vi "Test_Project Parser.vi"() -> ()   [LabVIEW 2019]
uses:
  Build/Project.Dependencies Finder.lvlibp/Dependency Source_VIPM/Dependency Source_VIPM.lvclass
  C:/Current projects/LV32.2019..ProjectDependenciesFinder/Build/Project.Dependencies Finder.lvlibp/Dependency Source/Dependency Source.lvclass
  Build/Project.Dependencies Finder.lvlibp/Dependency Source_NIPM/Dependency Source_NIPM.lvclass
  Build/Project.Dependencies Finder.lvlibp/Dependency Source_GPM/Dependency Source_GPM.lvclass
  Build/Project.Dependencies Finder.lvlibp/Dependency Source_Custom/Dependency Source_Custom.lvclass
  Build/Project.Dependencies Finder.lvlibp/Ctl/Ctl_Internal Target Element.ctl
  Build/Project.Dependencies Finder.lvlibp
  Build/Project.Dependencies Finder.lvlibp/Ctl/Ctl_External Target Element.ctl
  GPM/gpm_packages/@cs/actor-framework-messages/Source/MessageCycle/Message Cycle Notifications.ctl
  GPM/gpm_packages/@cs/actor-framework-messages/Source/MessageCycle/MessageCycle.lvclass
panel:
  in  "Load Stored Targets?(T)":bool=TRUE
  out "Unhandled Targets":string[](array[string])
  out "External Dependencies":string[](array[string])
  out "Internal Dependencies":string[](array[string])
  out "Error Out":errorcluster
  in  "Project Path in":path=path "C:/Current projects/LV32.2019..ProjectDependenciesFinder/_Test/Test.lvproj"
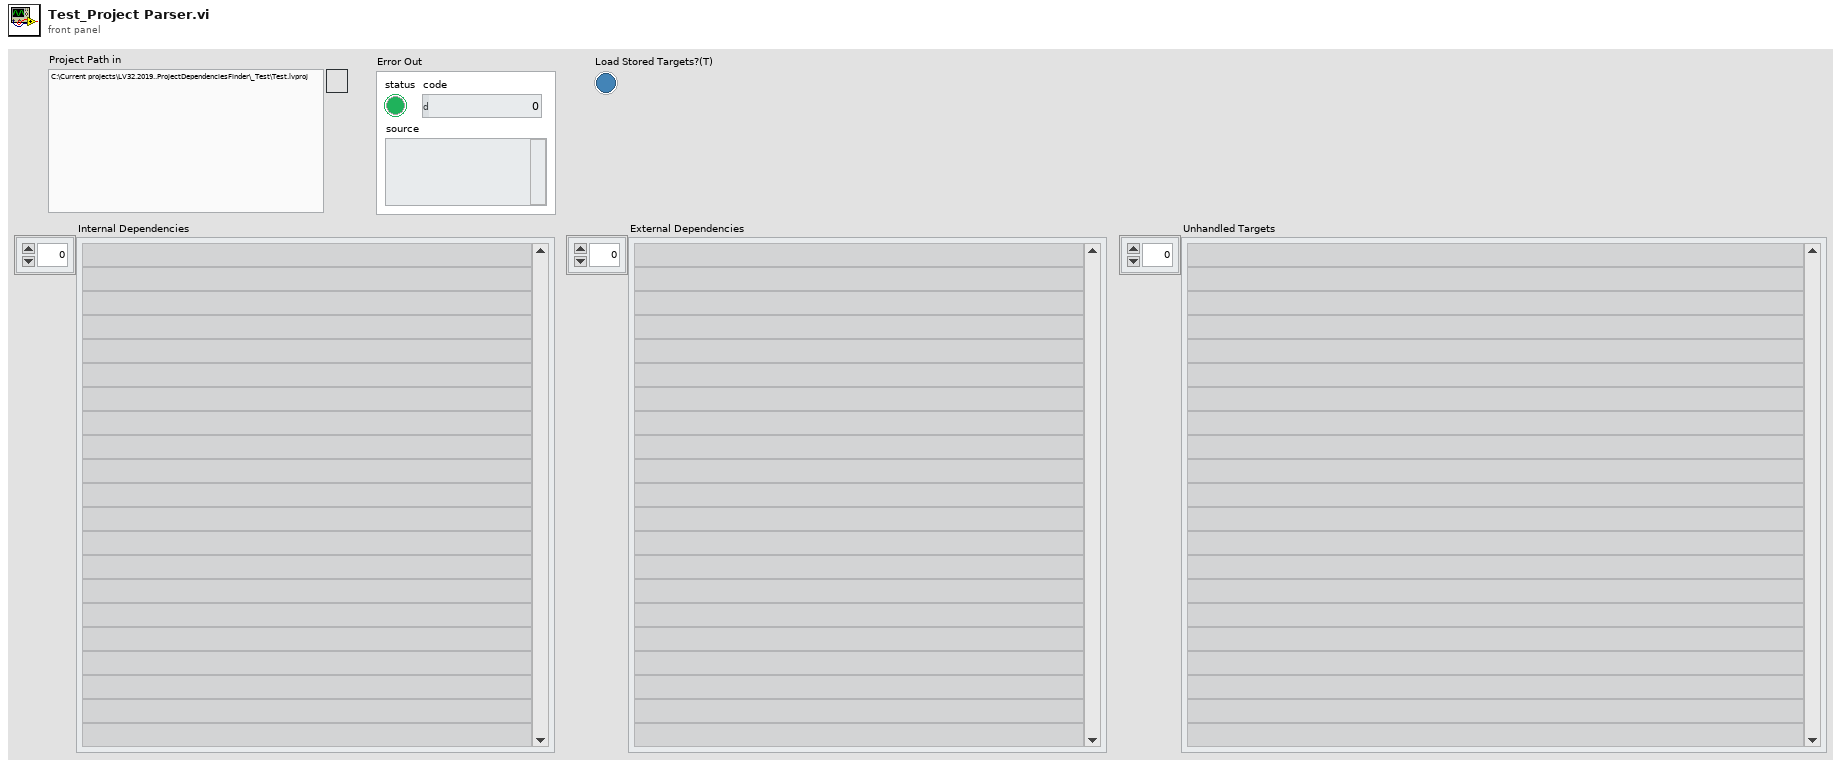
[diagram p1: front panel]
types:
  T1 = typedef "MessageCycle.lvclass/Message Cycle Notifications.ctl" = enum16{"Process Final Copy and Stop", "Stop Immediately", "Substitute Last Message and Stop"}
  T2 = typedef "Project.Dependencies Finder.lvlibp/Ctl_External Target Element.ctl" = cluster{"Target Source":string, "External Target Map":map{string, string}}
  T3 = typedef "Project.Dependencies Finder.lvlibp/Ctl_Internal Target Element.ctl" = cluster{"Target Source":string, "Internal Target Map":map{string, string}}
  T4 = typedef "Project.Dependencies Finder.lvlibp/Ctl_Dependency Element.ctl" = cluster{"Dependency Type":string, "Dependencies":string[]}
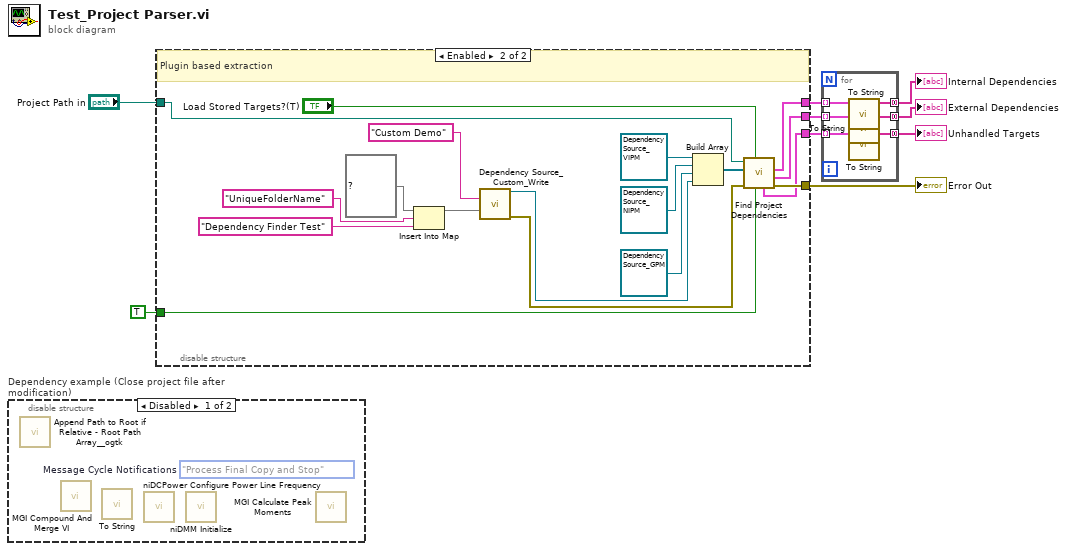
[diagram p0: block diagram]
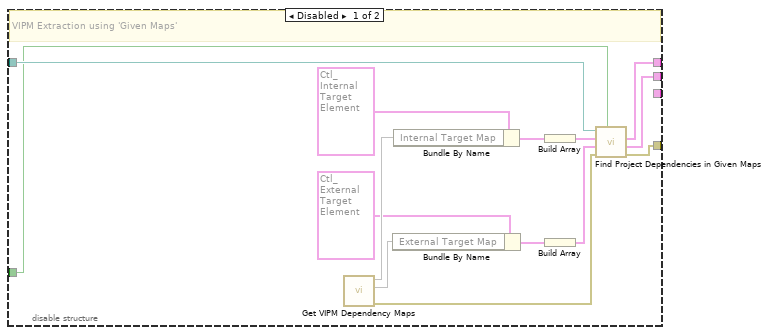
[diagram p2: hidden frame]
diagram:
  n1 = disable-structure "Dependency example (Close project file after modification)" shown="Disabled" {
    frame Disabled {
      (unwired) Message_Cycle_Notifications."Process Final Copy and Stop"  # Message Cycle Notifications
      n2 = call <userlib>:"Append Path to Root if Relative - Root Path Array__ogtk.vi"() -> ()  [unwired: 2 in, 1 out]
      n3 = call <userlib>:"MGI Compound And Merge VI.vi"() -> ()  [unwired: 1 in]
      n4 = call "To String.vi"() -> ()  [unwired: 11 in, 1 out]
      n5 = call <instrlib>:"niDCPower Configure Power Line Frequency.vi"() -> ()  [unwired: 10 in, 2 out]
      n6 = call <instrlib>:"niDMM Initialize.vi"() -> ()  [unwired: 10 in, 2 out]
      n7 = call <userlib>:"MGI Calculate Peak Moments.vi"() -> ()  [unwired: 3 in, 3 out]
    }
    frame Enabled {
    }
  }
  n8 = disable-structure shown="Enabled" {
    disable-tunnel: "Project Path in" -> [w23 w41]
    disable-tunnel: [w22 w38] -> w8
    disable-tunnel: [w18 w40] -> w7
    disable-tunnel: [w17 w39] -> w4
    disable-tunnel: TRUE ("To Lower Case?(T)") -> [w16 w32]
    disable-tunnel: [_ w35] -> w2
    frame Disabled {
      # "VIPM Extraction using 'Given Maps'"
      n9 = call "Get VIPM Dependency Maps.vi"() -> ("error out"=w10:errorcluster, "External Target Map"=w13:map{string, string}, "Internal Target Map"=w15:map{string, string})  [unwired: 7 in, 2 out]
      n10 = Bundle By Name(cluster=T2 {"Target Source"="VIPM", "External Target Map"={}} ("External Targets"), "External Target Map"=w13) -> (w12:T2)
      n11 = Bundle By Name(cluster=T3 {"Target Source"="VIPM", "Internal Target Map"={}} ("Internal Target Element"), "Internal Target Map"=w15) -> (w20:T3)
      n12 = Build Array(w20) -> (w19:T3[])
      n13 = Build Array(w12) -> (w11:T2[])
      n14 = call "Find Project Dependencies in Given Maps.vi"("To Lower Case?(T)"=w16, "Error In"=w10, "External Targets"=w11, "Internal Targets"=w19, "Project Path in"=w23) -> ("Error Out"=w22:errorcluster, "Found External Dependencies"=w17:T4[], "Found Internal Dependencies"=w18:T4[])  [unwired: 3 in, 1 out]
    }
    frame Enabled {
      # "Plugin based extraction"
      n15 = Insert Into Map(map in=map{string, string} {} ("External Target Map"), key="UniqueFolderName", value="Dependency Finder Test") -> (map out=w27:map{string, string})  [unwired: 2 out]
      n16 = call "Dependency Source_Custom_Write.vi"("Dependency Source Name"="Custom Demo", "External Target Map"=w27) -> ("Dependency Source_Custom out"=w30:refnum<class "Dependency Source_Custom.lvclass">, "error out"=w24:errorcluster)  [unwired: 12 in]
      n17 = Build Array(refnum<class "Dependency Source_VIPM.lvclass"> refnum ("Project.Dependencies Finder.lvlibp:Dependency Source_VIPM.lvclass"), refnum<class "Dependency Source_NIPM.lvclass"> refnum ("Project.Dependencies Finder.lvlibp:Dependency Source_NIPM.lvclass"), refnum<class "Dependency Source_GPM.lvclass"> refnum ("Project.Dependencies Finder.lvlibp:Dependency Source_GPM.lvclass"), w30) -> (w36:refnum<class "Dependency Source.lvclass">[])
      n18 = call "Find Project Dependencies.vi"("To Lower Case?(T)"=w32, "Load Stored Targets?(T)"="Load Stored Targets?(T)", "Error In"=w24, "Dependency Source Plugins"=w36, "Project Path in"=w41) -> ("Error Out"=w38:errorcluster, "Found External Dependencies"=w39:T4[], "Found Internal Dependencies"=w40:T4[], "Unhandled Targets"=w35:T4[])  [unwired: 1 in, 2 out]
    }
  }
  "Error Out" <- w8
  n19 = for {
    tunnel: w7 -> [w44] mode=indexing
    tunnel: [w47] -> w6 mode=concatenating
    tunnel: [w46] -> w5 mode=concatenating
    tunnel: w4 -> [w42] mode=indexing
    tunnel: w2 -> [w43] mode=indexing
    tunnel: [w45] -> w1 mode=concatenating
    n20 = call "To String.vi"("External Target Element"=w44) -> ("Dependencies"=w47:string[])  [unwired: 10 in]
    n21 = call "To String.vi"("External Target Element"=w42) -> ("Dependencies"=w46:string[])  [unwired: 10 in]
    n22 = call "To String.vi"("External Target Element"=w43) -> ("Dependencies"=w45:string[])  [unwired: 10 in]
  }
  "Internal Dependencies" <- w6
  "External Dependencies" <- w5
  "Unhandled Targets" <- w1
